vi "Async.Start.vi"(8 "error in (no error)":errorcluster, 11 "VS Inline Async API in":refnum<class "VS Inline Async API.lvclass">) -> (0 "error out":errorcluster, 3 "VS Inline Async API out":refnum<class "VS Inline Async API.lvclass">)   [LabVIEW 2015, in "VS Inline Async API.lvlib" / "VS Inline Async API.lvclass"]
uses:
  VS Inline Async API.lvclass
  VS Inline Async API.lvclass/VS Inline Async API.ctl
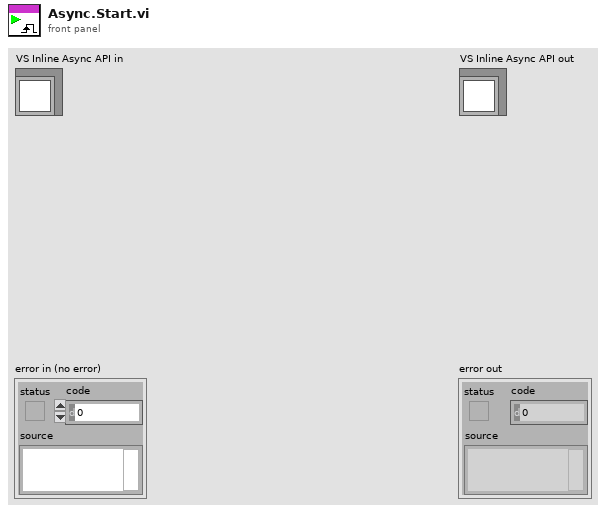
[diagram p1: front panel]
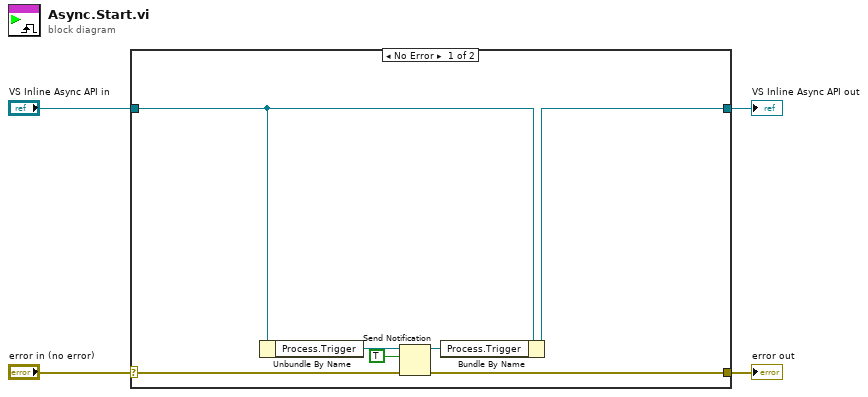
[diagram p0: block diagram]
diagram:
  n1 = case shown="No Error" "error in (no error)" {
    selector: "error in (no error)" -> [w7 w13]
    tunnel: [w6 w13] -> w3
    tunnel: [w10 w12] -> w1
    tunnel: "VS Inline Async API in" -> [w11 w12]
    frame No Error {
      n2 = Unbundle By Name(w11) -> ("Process.Trigger"=w9:refnum<notifier>)
      n3 = Send Notification(notification=TRUE, notifier=w9, error in (no error)=w7) -> (notifier out=w5:refnum<notifier>, error out=w6:errorcluster)
      n4 = Bundle By Name(cluster=w11, "Process.Trigger"=w5) -> (w10:refnum<class "VS Inline Async API.lvclass">)
    }
    frame Error {
    }
  }
  "error out" <- w3
  "VS Inline Async API out" <- w1
